vi "subSetParameters.vi"(10 "Rx Parameters":T2) -> (1 "Frame Parameters":T1={"IQ Rate"=0.0, "Frames"=0, "Length of Subset"=0, "Start Index of Subset"=0, "Start Carrier [Hz]"=88500000.0, "Stop Carrier [Hz]"=107700000.0, "Acq Duration [sec]"=0.01} {"Acq Duration [sec]" min=0.0 step=0.001 format="%#.6p"; "Stop Carrier [Hz]" min=50000000.0 max=6000000000.0 step=1000.0 format="%#.15p"; "Start Carrier [Hz]" min=50000000.0 max=6000000000.0 step=1000.0 format="%#.15p"}, 2 "test carrier frequencies":dbl[](array[numeric]), 3 "samples per acquisition":i32)   [LabVIEW 2017]
uses:
  subFrameParams.ctl
  <vilib>/Analysis/1siggen.llb/Ramp Pattern by Delta.vi
  <vilib>/Analysis/NI_AALBase.lvlib
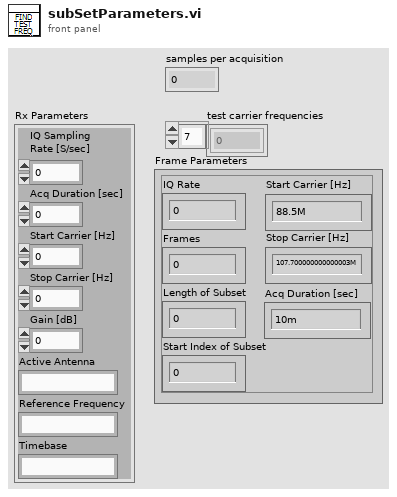
[diagram p1: front panel]
types:
  T1 = typedef "subFrameParams.ctl" = cluster{"IQ Rate":dbl, "Frames":i32, "Length of Subset":i32, "Start Index of Subset":i32, "Start Carrier [Hz]":dbl, "Stop Carrier [Hz]":dbl, "Acq Duration [sec]":dbl}
  T2 = cluster{"IQ Sampling\nRate [S/sec]":dbl, "Acq Duration [sec]":dbl, "Start Carrier [Hz]":dbl, "Stop Carrier [Hz]":dbl, "Gain [dB]":dbl, "Active Antenna":string, "Reference Frequency":string, "Timebase":string}
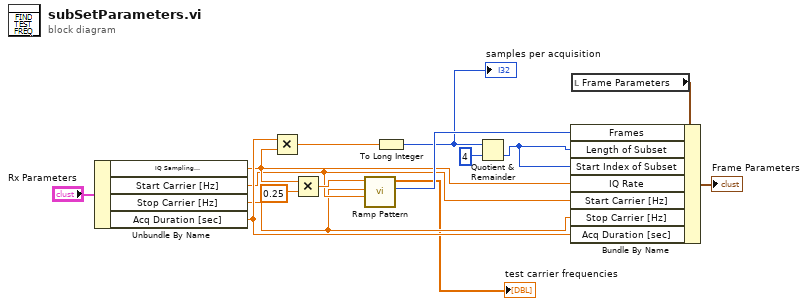
[diagram p0: block diagram]
diagram:
  n1 = Unbundle By Name("Rx Parameters") -> ("IQ Sampling\nRate [S/sec]"=w9:dbl, "Start Carrier [Hz]"=w8:dbl, "Stop Carrier [Hz]"=w7:dbl, "Acq Duration [sec]"=w10:dbl)
  n2 = Multiply(x=w10, y=w9) -> (x*y=w13:dbl)
  n3 = Multiply(x=w9, y=0.25) -> (x*y=w11:dbl)
  n4 = call-poly <vilib>:"Ramp Pattern.vi"("start"=w8, "end"=w7, "delta"=w11) -> ("samples"=w15:i32, "Ramp Pattern"=→"test carrier frequencies":dbl[])  [unwired: 6 in, 1 out]
  n5 = To Long Integer(number=w13) -> (32bit integer=w2:i32)
  "samples per acquisition" <- w2
  n6 = Quotient & Remainder(x=w2, y=4) -> (floor(x/y)=w1:i32)  [unwired: 1 out]
  n7 = local read "Frame Parameters"() -> (w4:T1)
  n8 = Bundle By Name(cluster=w4, "Frames"=w15, "Length of Subset"=w1, "Start Index of Subset"=w1, "IQ Rate"=w9, "Start Carrier [Hz]"=w8, "Stop Carrier [Hz]"=w7, "Acq Duration [sec]"=w10) -> (→"Frame Parameters":T1)
